vi "9219_FPGA_Temp.vi"(0 "FPGA VI Reference":T2, 5 "error in (no error)":errorcluster) -> (14 "Sensors":T1, 19 "error out":errorcluster)   [LabVIEW 2019]
uses:
  FPGA VI Ref.ctl
  C:/Program Files (x86)/National Instruments/LabVIEW 2019/examples/CompactRIO/Shared/cRIO Convert Thermocouple Readings.llb/Thermocouple Type.ctl
  <vilib>/Utility/error.llb/Error Cluster From Error Code.vi
  <vilib>/RVI Host/nirviSupport.llb/nirviErrorClusterFromErrorCode.vi
  <vilib>/rvi/errors/niLvFpgaAdjustHostInterfaceError.vi
  C:/Program Files (x86)/National Instruments/LabVIEW 2019/examples/CompactRIO/Module Specific/NI 9219/NI 9219 Scaling Utility/NI 9219 Scaling Support Files.llb/NI 9219 Convert Calibrated FXP to Thermocouple.vi
  <vilib>/rvi/interface/nirviMethod/nirviMethod.xnode
  <vilib>/rvi/interface/nirviReadWriteControl/nirviReadWriteControl.xnode
  <vilib>/FPGAPlugInAG/Dynamic/niLvFpga_AcknowledgeIrq_Dynamic.vi
  <vilib>/rvi/interface/nirviMethod/StockFPGA_InlinedMethodWaitForSingleIRQ.vi
  <vilib>/FPGAPlugInAG/Dynamic/niLvFpga_WaitOnIrq_Dynamic.vi
  NiFpgaLv.dll
  <vilib>/rvi/interface/Simulation/niFpgaSimulationCallBeginRW.vi
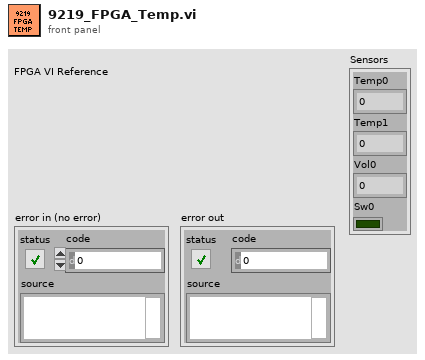
[diagram p1: front panel]
types:
  T1 = cluster{"Temp0":dbl, "Temp1":dbl, "Vol0":dbl, "Sw0":bool}
  T2 = typedef "FPGA VI Ref.ctl" = refnum<k20>
  T3 = typedef "Thermocouple Type.ctl" = u16
  T4 = cluster{"TC0":fxp<+/-,32,-1>, "CJC0":fxp<+/-,32,-1>, "Switch":bool, "RTD":fxp<+,32,14>, "Bridge":fxp<+/-,32,-1>}
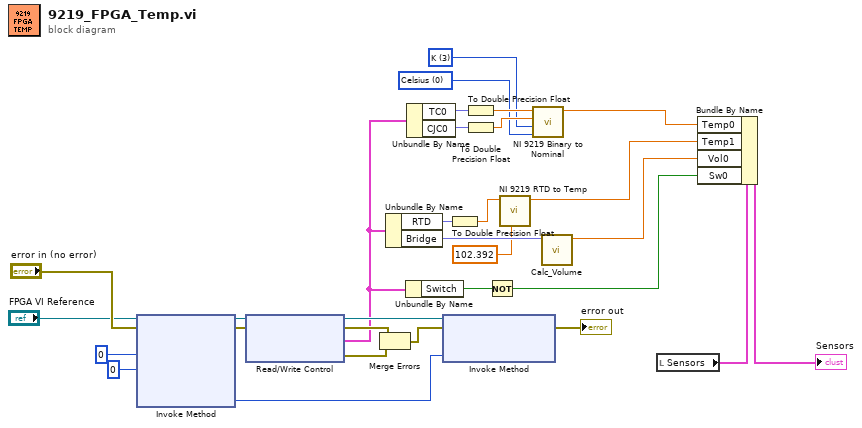
[diagram p0: block diagram]
diagram:
  w10 = T3 3 items=["B", "E", "J", "K", "R", "S", "T", "N"] ("CH1 ThermocoupleType")
  w11 = u16 0 items=["Celsius", "Fahrenheit", "Kelvin", "Rankine"] ("CH1 Temperature Units")
  n1 = xnode "Invoke Method"("FPGA VI Reference In"="FPGA VI Reference", "error in"="error in (no error)", "IRQ Number(s)"=0, "Timeout (ms)"=0 ("timeout (ms)(-1 for no timeout)")) -> ("FPGA VI Reference Out"=w12:T2, "error out"=w13:errorcluster, "IRQ(s) Asserted"=w14:i32)  [unwired: 1 out]
  n2 = xnode "Read/Write Control"("FPGA VI Reference In"=w12, "error in"=w13) -> ("FPGA VI Reference Out"=w15:T2, "error out"=w16:errorcluster, "9219 Output"=w3:T4, "FPGA Error Out"=w17:errorcluster)
  n3 = Merge Errors(w16, w17) -> (w18:errorcluster)
  n4 = Unbundle By Name(w3) -> ("RTD"=w7:fxp<+,32,14>, "Bridge"=w6:fxp<+/-,32,-1>)
  n5 = Unbundle By Name(w3) -> ("Switch"=w2:bool)
  n6 = Unbundle By Name(w3) -> ("TC0"=w19:fxp<+/-,32,-1>, "CJC0"=w20:fxp<+/-,32,-1>)
  n7 = xnode "Invoke Method"("FPGA VI Reference In"=w15, "error in"=w18, "IRQ Number(s)"=w14) -> ("error out"=→"error out":errorcluster)  [unwired: 1 out]
  n8 = To Double Precision Float(number=w7) -> (double precision float=w5:dbl)
  n9 = To Double Precision Float(number=w19) -> (double precision float=w21:dbl)
  n10 = To Double Precision Float(number=w20) -> (double precision float=w22:dbl)
  n11 = Not(x=w2) -> (.not. x?=w1:bool)
  n12 = call "NI 9219 RTD to Temp.vi"("Ro"=102.392, "RTD Resistance"=w5) -> ("RTDtemp"=w25:sgl)  [unwired: 8 in, 1 out]
  n13 = call-poly "NI 9219 Binary to Nominal.vi"("Temperature Units (C)"=w11, "ThermocoupleType"=w10, "CJC"=w22, "ADC Value"=w21) -> ("Temperature"=w26:dbl)  [unwired: 7 out]
  n14 = call "Calc_Volume.vi"("Bridge"=w6) -> ("Numeric"=w24:dbl)  [unwired: 10 in]
  n15 = local read "Sensors"() -> (w23:T1)
  n16 = Bundle By Name(cluster=w23, "Temp0"=w26, "Temp1"=w25, "Vol0"=w24, "Sw0"=w1) -> (→"Sensors":T1)
